vi "Com_Cmd_RevA.vi"(6 "Timeout":i32=10000, 7 "Query":bool, 8 "error in":errorcluster, 9 "Delay, ms":u32=1000, 10 "write buffer":string="PM:P?", 11 "VISA":refnum<visa-resource-name>="COM1") -> (0 "error out":errorcluster, 1 "number":dbl format="%#.6e", 2 "read buffer":string, 3 "VISA Out":refnum<visa-resource-name>, 4 "Timeout":bool, 5 "return count":u32)   [LabVIEW 2017]
panel:
  out "Retry Attempts":i32
  in  "Max Retries for COM port":i32=10
  out "Temp Buffer":string
  out "old buffer":string
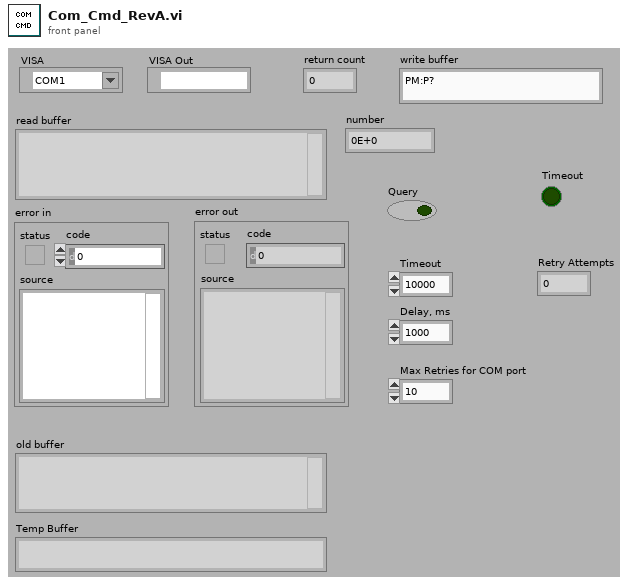
[diagram p1: front panel]
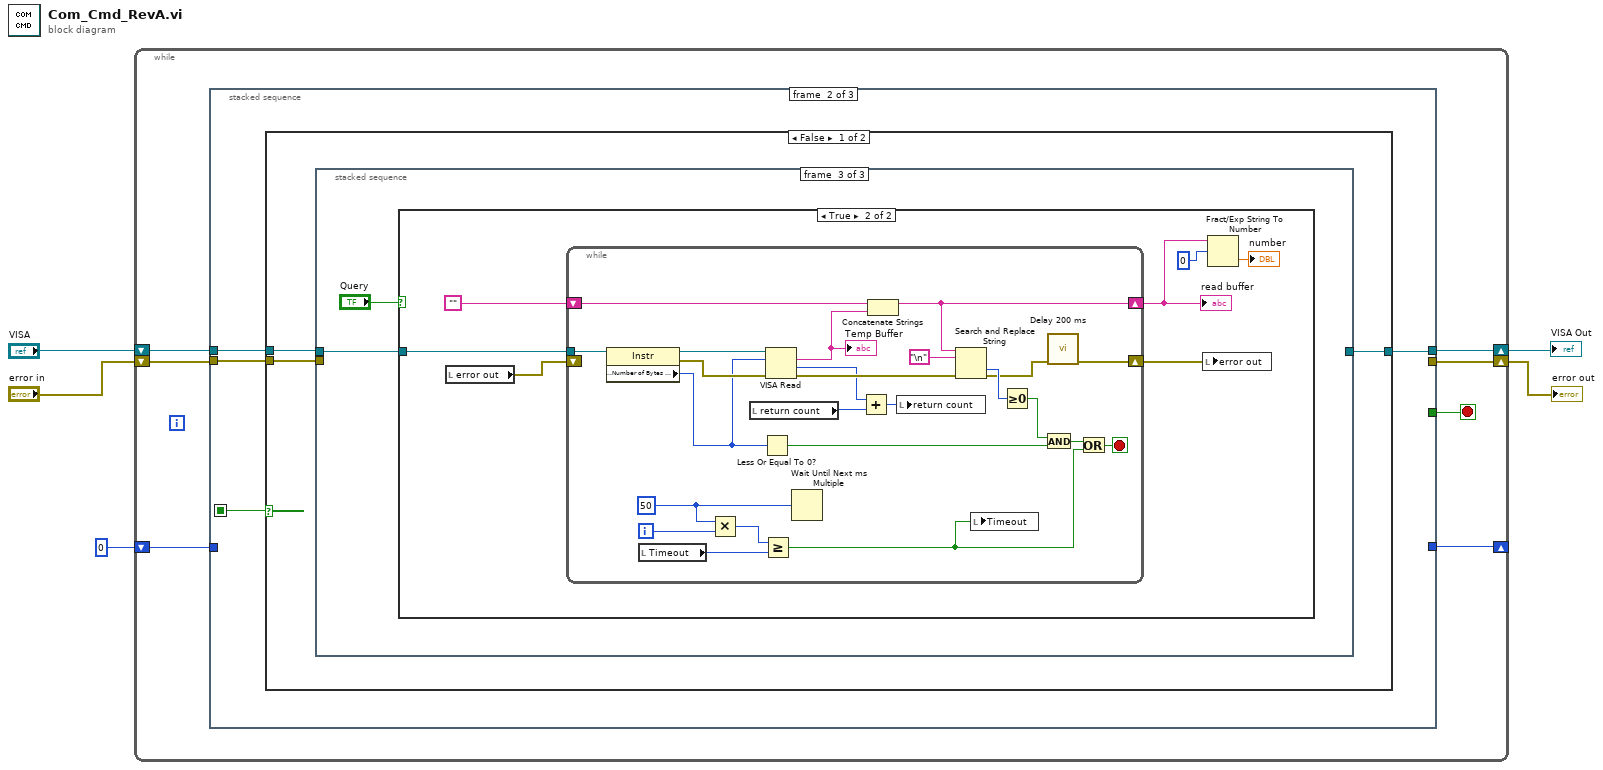
[diagram p0: block diagram]
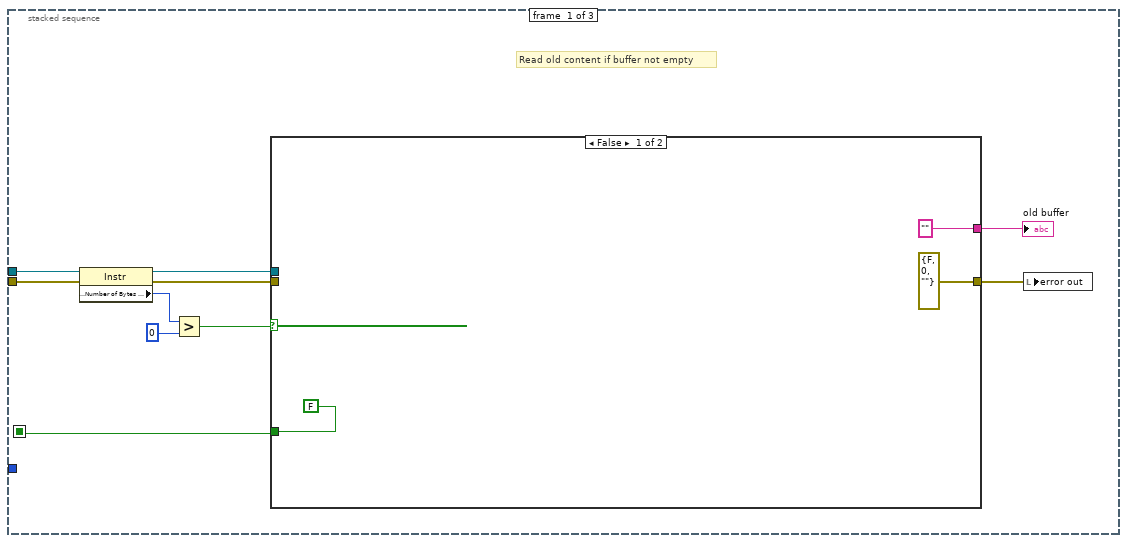
[diagram p2: hidden frame]
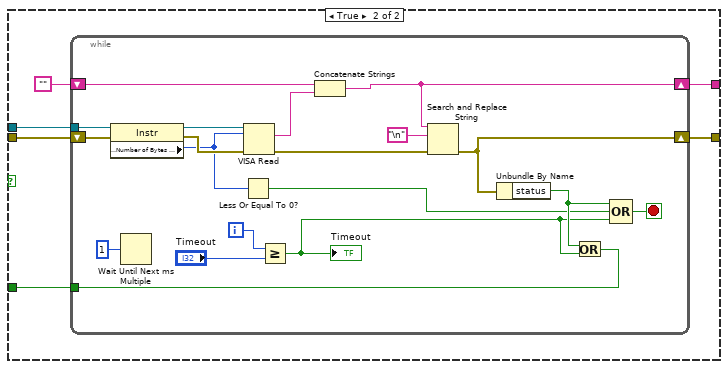
[diagram p3: hidden frame]
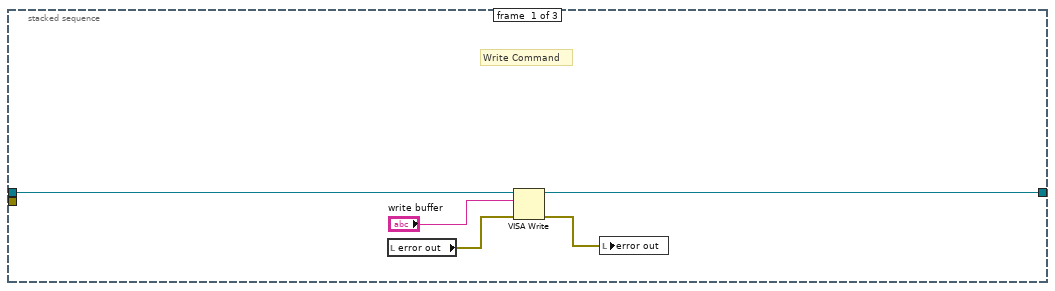
[diagram p4: hidden frame]
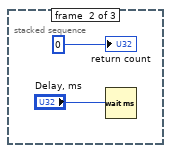
[diagram p5: hidden frame]
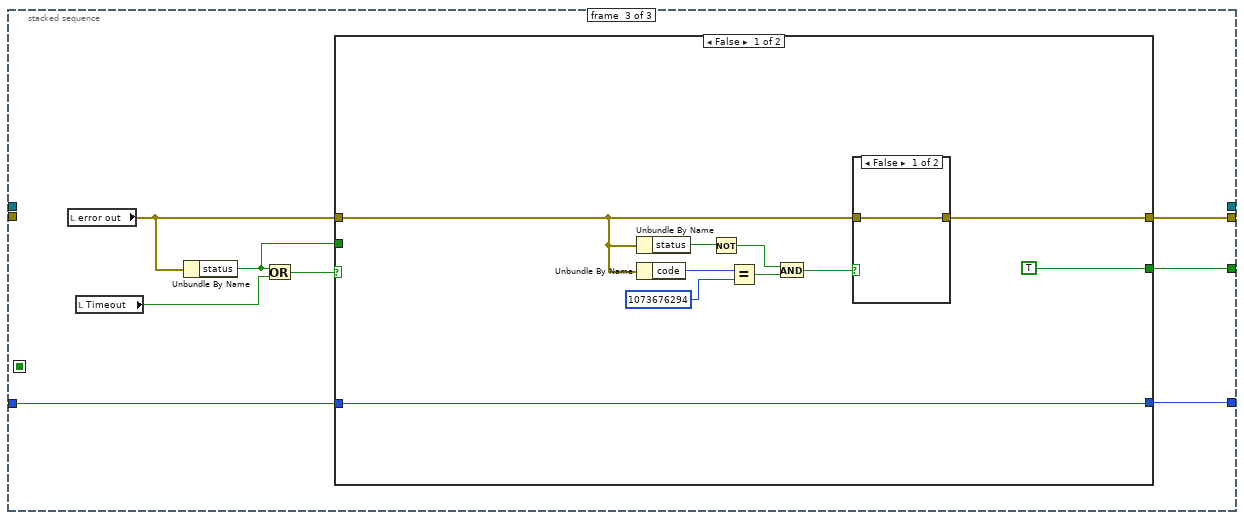
[diagram p8: hidden frame]
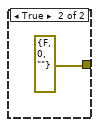
[diagram p9: hidden frame]
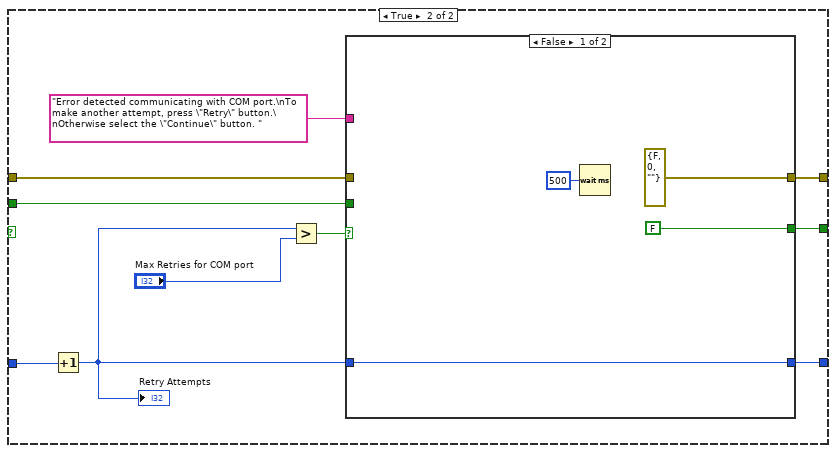
[diagram p10: hidden frame]
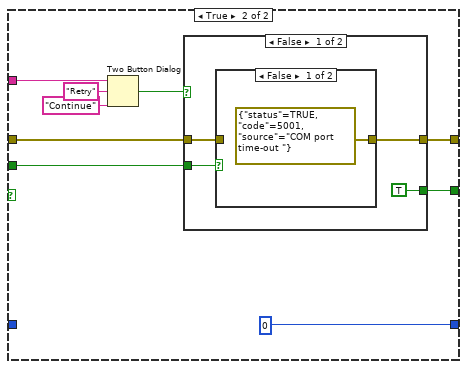
[diagram p11: hidden frame]
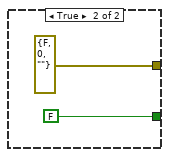
[diagram p13: hidden frame]
diagram:
  n1 = while {
    shift-right: [w10] -> w3
    shift-left: "VISA" -> [w12]
    shift-right: [w9] -> w2
    shift-left: "error in" -> [w11]
    shift-right: [w6] -> _
    shift-left: 0 -> [w7]
    stop <- w8 stop-if-true
    n2 = stacked-sequence {
      seq-local: [w16 _ _] -> [_ w54 _]
      tunnel: w11 -> [w17 w53 _]
      tunnel: w12 -> [w15 w52 _]
      tunnel: [_ w51 _] -> w10
      tunnel: [_ _ w103] -> w9
      tunnel: [_ _ w102] -> w8
      tunnel: w7 -> [_ _ w101]
      tunnel: [_ _ w100] -> w6
      frame #0 {
        # "Read old content if buffer not empty"
        n3 = property class="Instr"(reference=w15, error in=w17) -> (reference out=w19:refnum<visa-resource-name>, error out=w20:errorcluster, "Serial Settings:Number of Bytes at Serial Port"=w21:u32)
        n4 = Greater?(x=w21, y=u32 0) -> (0:w18:bool)
        n5 = case shown="False" w18 {
          tunnel: w20 -> [_ w29]
          tunnel: w19 -> [_ w31]
          tunnel: [FALSE ("Timeout") w28] -> w16
          tunnel: ["" w27] -> w14
          tunnel: [errorcluster {"status"=FALSE, "code"=0, "source"=""} ("error out") w26] -> w13
          frame False {
          }
          frame True {
            n6 = while {
              tunnel: w31 -> [w41]
              shift-right: [w47] -> w27
              shift-left: "" -> [w49]
              shift-right: [w36] -> w26
              shift-left: w29 -> [w38]
              tunnel: [w33] -> w28
              i -> [w45]
              stop <- w44 stop-if-true
              n7 = property class="Instr"(reference=w41, error in=w38) -> (reference out=w43:refnum<visa-resource-name>, error out=w42:errorcluster, "Serial Settings:Number of Bytes at Serial Port"=w39:u32)
              n8 = Wait Until Next ms Multiple(millisecond multiple=u32 1) -> ()  [unwired: 1 out]
              n9 = Less Or Equal To 0?(x=w39) -> (x <= 0?=w34:bool)
              n10 = VISA Read(VISA resource name=w43, byte count=w39, error in (no error)=w42) -> (read buffer=w48:string, error out=w46:errorcluster)  [unwired: 2 out]
              n11 = Greater Or Equal?(x=w45, y="Timeout") -> (x >= y?=w32:bool)
              "Timeout" <- w32
              n12 = Concatenate Strings(w49, w48) -> (w47:string)
              n13 = Search and Replace String(input string=w47, search string="\n", error in=w46) -> (error out=w36:errorcluster)  [unwired: 5 in, 3 out]
              n14 = Unbundle By Name(w36) -> ("status"=w35:bool)
              n15 = Or(x=w35, y=w32) -> (x .or. y?=w33:bool)
              n16 = Compound Arithmetic op=OR(w35, w34, w32) -> (w44:bool)
            }
          }
        }
        "old buffer" <- w14
        n17 = local write "error out"(w13) -> ()
      }
      frame #1 {
        n18 = case shown="False" w54 {
          tunnel: w53 -> [w57 _]
          tunnel: w52 -> [w56 w98]
          tunnel: [w55 w98] -> w51
          frame False {
            n19 = stacked-sequence {
              tunnel: w56 -> [w59 _ w65]
              tunnel: w57 -> [_ _ _]
              tunnel: [w58 _ _] -> w55
              frame #0 {
                # "Write Command"
                n20 = local read "error out"() -> (w61:errorcluster)
                n21 = VISA Write(VISA resource name=w59, write buffer="write buffer", error in (no error)=w61) -> (VISA resource name out=w58:refnum<visa-resource-name>, error out=w62:errorcluster)  [unwired: 1 out]
                n22 = local write "error out"(w62) -> ()
              }
              frame #1 {
                n23 = Wait (ms)(milliseconds to wait="Delay, ms") -> ()  [unwired: 1 out]
                "return count" <- u32 0 ("return count")
              }
              frame #2 {
                n24 = case shown="True" "Query" {
                  tunnel: w65 -> [_ w69]
                  frame False {
                  }
                  frame True {
                    n25 = local read "error out"() -> (w67:errorcluster)
                    n26 = while {
                      tunnel: w69 -> [w79]
                      shift-right: [w87] -> w71
                      shift-left: "" -> [w97]
                      shift-right: [w74] -> w68
                      shift-left: w67 -> [_]
                      i -> [w81]
                      stop <- w94 stop-if-true
                      w78 = 50
                      n27 = property class="Instr"(reference=w79) -> (reference out=w93:refnum<visa-resource-name>, error out=w92:errorcluster, "Serial Settings:Number of Bytes at Serial Port"=w91:u32)  [unwired: 1 in]
                      n28 = local read "Timeout"() -> (w95:i32)
                      n29 = Multiply(x=w78, y=w81) -> (x*y=w80:i32)
                      n30 = local read "return count"() -> (w84:u32)
                      n31 = Less Or Equal To 0?(x=w91) -> (x <= 0?=w89:bool)
                      n32 = Greater Or Equal?(x=w80, y=w95) -> (x >= y?=w76:bool)
                      n33 = VISA Read(VISA resource name=w93, byte count=w91, error in (no error)=w92) -> (read buffer=w86:string, return count=w85:u32, error out=w96:errorcluster)  [unwired: 1 out]
                      "Temp Buffer" <- w86
                      n34 = Wait Until Next ms Multiple(millisecond multiple=w78) -> ()  [unwired: 1 out]
                      n35 = Add(x=w85, y=w84) -> (x+y=w83:u32)
                      n36 = Concatenate Strings(w97, w86) -> (w87:string)
                      n37 = local write "return count"(w83) -> ()
                      n38 = Search and Replace String(input string=w87, search string="\n", error in=w96) -> (offset past replacement=w88:i32, error out=w75:errorcluster)  [unwired: 5 in, 2 out]
                      n39 = local write "Timeout"(w76) -> ()
                      n40 = Greater Or Equal To 0?(x=w88) -> (x >= 0?=w90:bool)
                      n41 = And(x=w90, y=w89) -> (x .and. y?=w77:bool)
                      n42 = call "Delay 200 ms"("error in (no error)"=w75) -> ("error out"=w74:errorcluster)  [unwired: 10 in]
                      n43 = Or(x=w77, y=w76) -> (x .or. y?=w94:bool)
                    }
                    "read buffer" <- w71
                    n44 = local write "error out"(w68) -> ()
                    n45 = Fract/Exp String To Number(string=w71, offset=0) -> (number=→"number":dbl)  [unwired: 2 in, 1 out]
                  }
                }
              }
            }
          }
          frame True {
          }
        }
      }
      frame #2 {
        n46 = local read "error out"() -> (w104:errorcluster)
        n47 = local read "Timeout"() -> (w105:bool)
        n48 = Unbundle By Name(w104) -> ("status"=w99:bool)
        n49 = Or(x=w99, y=w105) -> (x .or. y?=w106:bool)
        n50 = case shown="False" w106 {
          tunnel: w104 -> [w110 w128]
          tunnel: [w109 w127] -> w103
          tunnel: [TRUE w126] -> w102
          tunnel: w101 -> [w107 w124]
          tunnel: [w107 w121] -> w100
          tunnel: w99 -> [_ w119]
          frame False {
            n51 = Unbundle By Name(w110) -> ("status"=w115:bool)
            n52 = Unbundle By Name(w110) -> ("code"=w116:i32)
            n53 = Not(x=w115) -> (.not. x?=w113:bool)
            n54 = Equal?(x=w116, y=1073676294) -> (x = y?=w114:bool)
            n55 = And(x=w113, y=w114) -> (x .and. y?=w112:bool)
            n56 = case shown="False" w112 {
              tunnel: [w117 errorcluster {"status"=FALSE, "code"=0, "source"=""} ("error out")] -> w109
              tunnel: w110 -> [w117 _]
              frame False {
              }
              frame True {
              }
            }
          }
          frame True {
            n57 = Increment(x=w124) -> (x+1=w120:i32)
            "Retry Attempts" <- w120
            n58 = Greater?(x=w120, y="Max Retries for COM port") -> (0:w122:bool)
            n59 = case shown="False" w122 {
              tunnel: [errorcluster {"status"=FALSE, "code"=0, "source"=""} ("error out") w136] -> w127
              tunnel: w128 -> [_ w135]
              tunnel: [FALSE w141] -> w126
              tunnel: "Error detected communicating with COM port.\nTo make another attempt, press \"Retry\" button.\nOtherwise select the \"Continue\" button. " ("message") -> [_ w140]
              tunnel: [w129 0] -> w121
              tunnel: w120 -> [w129 _]
              tunnel: w119 -> [_ w133]
              frame False {
                n60 = Wait (ms)(milliseconds to wait=u32 500) -> ()  [unwired: 1 out]
              }
              frame True {
                n61 = Two Button Dialog(message=w140, 1:"Continue" ("F button name (\"Cancel\")"), 2:"Retry" ("T button name (\"OK\")")) -> (T button?=w137:bool)
                n62 = case shown="False" w137 {
                  tunnel: [TRUE FALSE] -> w141
                  tunnel: [w142 errorcluster {"status"=FALSE, "code"=0, "source"=""} ("error out")] -> w136
                  tunnel: w135 -> [w143 _]
                  tunnel: w133 -> [w144 _]
                  frame False {
                    n63 = case shown="False" w144 {
                      tunnel: [errorcluster {"status"=TRUE, "code"=5001, "source"="COM port time-out "} ("error constant") w147] -> w142
                      tunnel: w143 -> [_ w147]
                      frame False {
                      }
                      frame True {
                      }
                    }
                  }
                  frame True {
                  }
                }
              }
            }
          }
        }
      }
    }
  }
  "error out" <- w2
  "VISA Out" <- w3
